vi "Create Half-H Command.vi"(8 "error in (no error)":errorcluster, 11 "Section Ptr":T8 format="%.0x") -> (0 "error out":errorcluster, 3 "Parent Ref out":T8 format="%.0x")   [LabVIEW 2015, in "DCM System Explorer.lvlib"]
uses:
  DCM System Explorer.lvlib
  <vilib>/NI Veristand/Custom Device API/Custom Device Item Ref.ctl
  <vilib>/Powertrain Controls/Device Drivers/DCM/HH/RT/Setup.ctl
  <vilib>/Powertrain Controls/Device Drivers/DCM/HH/FPGA/Mode.ctl
  <vilib>/Powertrain Controls/Device Drivers/DCM/Rev0/FPGA/Digital Channel.ctl
  <vilib>/Powertrain Controls/Device Drivers/DCM/HH/RT/Angle Control.ctl
  <vilib>/Powertrain Controls/Device Drivers/DCM/HH/RT/Config.ctl
  <vilib>/Powertrain Controls/Device Drivers/DCM/HH/RT/Mode.ctl
  <vilib>/Powertrain Controls/Device Drivers/DCM/HH/RT/ISeq.ctl
  <vilib>/NI Veristand/Custom Device API/Custom Device Channel Type.ctl
  Shared/DCM Constants and GUIDs.vi
  Shared/DCM Properties.vi
  <vilib>/NI VeriStand/Custom Device API/Custom Device API.lvlib
  DCM Shared.lvlib
  <vilib>/Powertrain Controls/Device Drivers/DCM/HH/RT/DCM - RT - HH.lvlib
  <vilib>/Powertrain Controls/Device Drivers/DCM/Rev0/FPGA/DCM - FPGA.lvlib
  <vilib>/Powertrain Controls/Device Drivers/DCM/HH/FPGA/DCM - FPGA - HH.lvlib
panel:
  in  "Config":T1[](array[typedef]) {"ISeq"."Duration [s]" min=0 max=26 format="%#_3p"; "ISeq"."Lower [A]" min=0 max=8 format="%#_3p"; "ISeq"."Upper [A]" min=0 max=8 format="%#_3p"}
  in  "Command":T4[](array[typedef])=[{"Mode"=enum."Off", "Digital Input"=enum."Unused", "Polarity"=FALSE, "Frequency [Hz]"=0.0, "Duty Cycle [%]"=0.0, "TDC Offset [CAD]"=0.0, "Window Start [DBTDC]"=0.0, "Window End [DBTDC]"=0.0, "Angles"=[{"Enable"=FALSE, "Location [DBTDC]"=0.0, "Duration [s]"=0.0}, {"Enable"=FALSE, "Location [DBTDC]"=0.0, "Duration [s]"=0.0}, {"Enable"=FALSE, "Location [DBTDC]"=0.0, "Duration [s]"=0.0}, {"Enable"=FALSE, "Location [DBTDC]"=0.0, "Duration [s]"=0.0}], "Skip Fire"=FALSE, "Skip Fire Index"=0}, {"Mode"=enum."Off", "Digital Input"=enum."Unused", "Polarity"=FALSE, "Frequency [Hz]"=0.0, "Duty Cycle [%]"=0.0, "TDC Offset [CAD]"=0.0, "Window Start [DBTDC]"=0.0, "Window End [DBTDC]"=0.0, "Angles"=[{"Enable"=FALSE, "Location [DBTDC]"=0.0, "Duration [s]"=0.0}, {"Enable"=FALSE, "Location [DBTDC]"=0.0, "Duration [s]"=0.0}, {"Enable"=FALSE, "Location [DBTDC]"=0.0, "Duration [s]"=0.0}, {"Enable"=FALSE, "Location [DBTDC]"=0.0, "Duration [s]"=0.0}], "Skip Fire"=FALSE, "Skip Fire Index"=0}, {"Mode"=enum."Off", "Digital Input"=enum."Unused", "Polarity"=FALSE, "Frequency [Hz]"=0.0, "Duty Cycle [%]"=0.0, "TDC Offset [CAD]"=0.0, "Window Start [DBTDC]"=0.0, "Window End [DBTDC]"=0.0, "Angles"=[{"Enable"=FALSE, "Location [DBTDC]"=0.0, "Duration [s]"=0.0}, {"Enable"=FALSE, "Location [DBTDC]"=0.0, "Duration [s]"=0.0}, {"Enable"=FALSE, "Location [DBTDC]"=0.0, "Duration [s]"=0.0}, {"Enable"=FALSE, "Location [DBTDC]"=0.0, "Duration [s]"=0.0}], "Skip Fire"=FALSE, "Skip Fire Index"=0}, {"Mode"=enum."Off", "Digital Input"=enum."Unused", "Polarity"=FALSE, "Frequency [Hz]"=0.0, "Duty Cycle [%]"=0.0, "TDC Offset [CAD]"=0.0, "Window Start [DBTDC]"=0.0, "Window End [DBTDC]"=0.0, "Angles"=[{"Enable"=FALSE, "Location [DBTDC]"=0.0, "Duration [s]"=0.0}, {"Enable"=FALSE, "Location [DBTDC]"=0.0, "Duration [s]"=0.0}, {"Enable"=FALSE, "Location [DBTDC]"=0.0, "Duration [s]"=0.0}, {"Enable"=FALSE, "Location [DBTDC]"=0.0, "Duration [s]"=0.0}], "Skip Fire"=FALSE, "Skip Fire Index"=0}, {"Mode"=enum."Off", "Digital Input"=enum."Unused", "Polarity"=FALSE, "Frequency [Hz]"=0.0, "Duty Cycle [%]"=0.0, "TDC Offset [CAD]"=0.0, "Window Start [DBTDC]"=0.0, "Window End [DBTDC]"=0.0, "Angles"=[{"Enable"=FALSE, "Location [DBTDC]"=0.0, "Duration [s]"=0.0}, {"Enable"=FALSE, "Location [DBTDC]"=0.0, "Duration [s]"=0.0}, {"Enable"=FALSE, "Location [DBTDC]"=0.0, "Duration [s]"=0.0}, {"Enable"=FALSE, "Location [DBTDC]"=0.0, "Duration [s]"=0.0}], "Skip Fire"=FALSE, "Skip Fire Index"=0}, {"Mode"=enum."Off", "Digital Input"=enum."Unused", "Polarity"=FALSE, "Frequency [Hz]"=0.0, "Duty Cycle [%]"=0.0, "TDC Offset [CAD]"=0.0, "Window Start [DBTDC]"=0.0, "Window End [DBTDC]"=0.0, "Angles"=[{"Enable"=FALSE, "Location [DBTDC]"=0.0, "Duration [s]"=0.0}, {"Enable"=FALSE, "Location [DBTDC]"=0.0, "Duration [s]"=0.0}, {"Enable"=FALSE, "Location [DBTDC]"=0.0, "Duration [s]"=0.0}, {"Enable"=FALSE, "Location [DBTDC]"=0.0, "Duration [s]"=0.0}], "Skip Fire"=FALSE, "Skip Fire Index"=0}, {"Mode"=enum."Off", "Digital Input"=enum."Unused", "Polarity"=FALSE, "Frequency [Hz]"=0.0, "Duty Cycle [%]"=0.0, "TDC Offset [CAD]"=0.0, "Window Start [DBTDC]"=0.0, "Window End [DBTDC]"=0.0, "Angles"=[{"Enable"=FALSE, "Location [DBTDC]"=0.0, "Duration [s]"=0.0}, {"Enable"=FALSE, "Location [DBTDC]"=0.0, "Duration [s]"=0.0}, {"Enable"=FALSE, "Location [DBTDC]"=0.0, "Duration [s]"=0.0}, {"Enable"=FALSE, "Location [DBTDC]"=0.0, "Duration [s]"=0.0}], "Skip Fire"=FALSE, "Skip Fire Index"=0}, {"Mode"=enum."Off", "Digital Input"=enum."Unused", "Polarity"=FALSE, "Frequency [Hz]"=0.0, "Duty Cycle [%]"=0.0, "TDC Offset [CAD]"=0.0, "Window Start [DBTDC]"=0.0, "Window End [DBTDC]"=0.0, "Angles"=[{"Enable"=FALSE, "Location [DBTDC]"=0.0, "Duration [s]"=0.0}, {"Enable"=FALSE, "Location [DBTDC]"=0.0, "Duration [s]"=0.0}, {"Enable"=FALSE, "Location [DBTDC]"=0.0, "Duration [s]"=0.0}, {"Enable"=FALSE, "Location [DBTDC]"=0.0, "Duration [s]"=0.0}], "Skip Fire"=FALSE, "Skip Fire Index"=0}] {"Skip Fire Index" max=7; "Angles"."Duration [s]" format="%#_3p"; "Frequency [Hz]" format="%#_3p"}
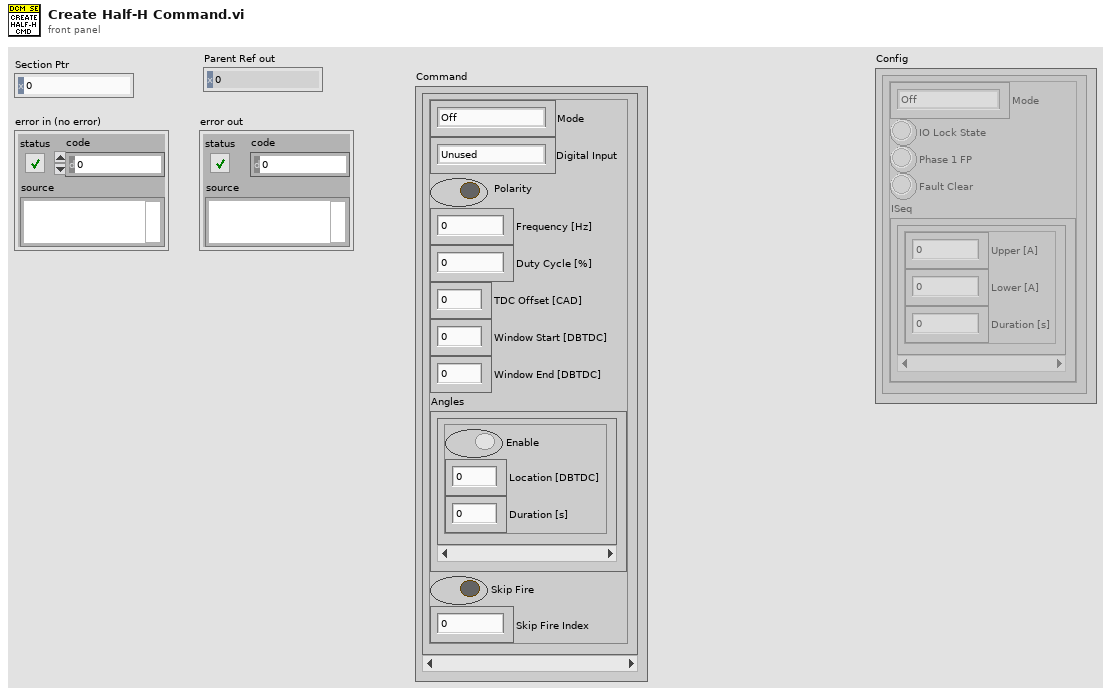
[diagram p1: front panel]
types:
  T1 = typedef "DCM - RT - HH.lvlib/Config.ctl" = cluster{"Mode":T2, "IO Lock State":bool, "Phase 1 FP":bool, "Fault Clear":bool, "ISeq":T3[]}
  T2 = typedef "DCM - RT - HH.lvlib/Mode.ctl" = enum16{"Off", "Lowside", "Highside", "PFI", "Full H", "3-Phase"}
  T3 = typedef "DCM - RT - HH.lvlib/ISeq.ctl" = cluster{"Upper [A]":sgl, "Lower [A]":sgl, "Duration [s]":sgl}
  T4 = typedef "DCM - RT - HH.lvlib/Setup.ctl" = cluster{"Mode":T5, "Digital Input":T6, "Polarity":bool, "Frequency [Hz]":sgl, "Duty Cycle [%]":sgl, "TDC Offset [CAD]":sgl, "Window Start [DBTDC]":sgl, "Window End [DBTDC]":sgl, "Angles":T7[], "Skip Fire":bool, "Skip Fire Index":u8}
  T5 = typedef "DCM - FPGA - HH.lvlib/Mode.ctl" = enum8{"Off", "Direct", "Pulse Width Modulation", "Engine Position Tracking"}
  T6 = typedef "DCM - FPGA.lvlib/Digital Channel.ctl" = enum8{"Unused", "Diff IO 1", "Diff IO 2", "Diff IO 3", "Diff IO 4", "Diff IO 5", "Diff IO 6", "Diff IO 7", "Diff IO 8", "Aux 1", "Aux 2", "Aux 3", "Aux 4", "Aux 5", "Aux 6", "Aux 7", "Aux 8", "User OS"}
  T7 = typedef "DCM - RT - HH.lvlib/Angle Control.ctl" = cluster{"Enable":bool, "Location [DBTDC]":sgl, "Duration [s]":sgl}
  T8 = typedef "Custom Device API.lvlib/Custom Device Item Ref.ctl" = u64
  T9 = typedef "Custom Device API.lvlib/Custom Device Channel Type.ctl" = enum16{"Input", "Output"}
  T10 = typedef "DCM Shared.lvlib/Channel.ctl" = cluster{"Name":string, "Units":string, "Default":dbl, "Description":string}
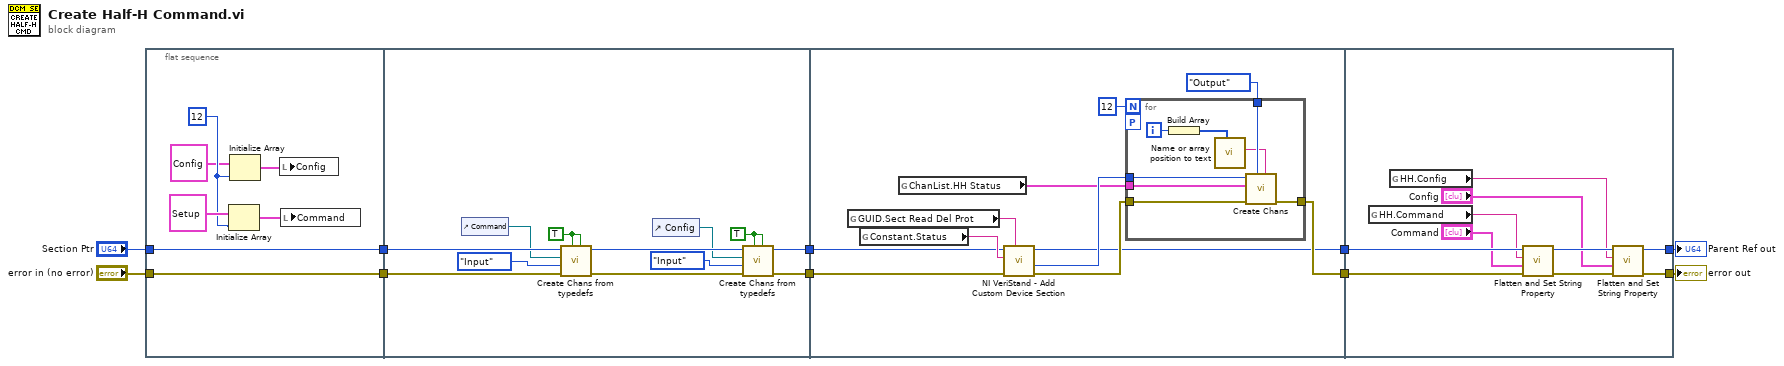
[diagram p0: block diagram]
diagram:
  n1 = flat-sequence {
    tunnel: [w16] -> w8
    tunnel: [w17] -> w9
    tunnel: "error in (no error)" -> [w17]
    tunnel: "Section Ptr" -> [w16]
    tunnel: [w23] -> w2
    tunnel: w9 -> [w20]
    tunnel: w8 -> [w21]
    tunnel: [w22] -> w4
    tunnel: w4 -> [w33]
    tunnel: [w30] -> w3
    tunnel: w2 -> [w32]
    tunnel: [w31] -> w1
    tunnel: [w49] -> w10
    tunnel: [w50] -> w5
    tunnel: w3 -> [w57]
    tunnel: w1 -> [w58]
    frame #0 {
      w13 = 12 ("dimension size")
      n2 = Initialize Array(T4 {"Mode"=enum."Off", "Digital Input"=enum."Unused", "Polarity"=FALSE, "Frequency [Hz]"=0.0, "Duty Cycle [%]"=0.0, "TDC Offset [CAD]"=0.0, "Window Start [DBTDC]"=0.0, "Window End [DBTDC]"=0.0, "Angles"=[{"Enable"=FALSE, "Location [DBTDC]"=0.0, "Duration [s]"=0.0}, {"Enable"=FALSE, "Location [DBTDC]"=0.0, "Duration [s]"=0.0}, {"Enable"=FALSE, "Location [DBTDC]"=0.0, "Duration [s]"=0.0}, {"Enable"=FALSE, "Location [DBTDC]"=0.0, "Duration [s]"=0.0}], "Skip Fire"=FALSE, "Skip Fire Index"=0}, w13) -> (w14:T4[])
      n3 = Initialize Array(T1 {"Mode"=enum."Off", "IO Lock State"=FALSE, "Phase 1 FP"=FALSE, "Fault Clear"=FALSE, "ISeq"=[{"Upper [A]"=0.0, "Lower [A]"=0.0, "Duration [s]"=0.0}, {"Upper [A]"=0.0, "Lower [A]"=0.0, "Duration [s]"=0.0}, {"Upper [A]"=0.0, "Lower [A]"=0.0, "Duration [s]"=0.0}, {"Upper [A]"=0.0, "Lower [A]"=0.0, "Duration [s]"=0.0}]} ("HH Config"), w13) -> (w11:T1[])
      n4 = local write "Config"(w11) -> ()
      n5 = local write "Command"(w14) -> ()
    }
    frame #1 {
      w27 = TRUE ("Prevent overwrite? (F)")
      w28 = TRUE ("Prevent overwrite? (F)")
      n6 = control-ref of="Command"() -> (w18:refnum<vi>)
      n7 = call "Create Chans from typedefs.vi"("Default from text? (F)"=w28, "Prevent overwrite? (F)"=w28, "error in"=w20, "Type"=Custom_Device_Channel_Type."Input", "Ctl Ref"=w18, "Section Ref in"=w21) -> ("error out"=w24:errorcluster, "Section Ref out"=w25:T8)  [unwired: 3 in, 1 out]
      n8 = control-ref of="Config"() -> (w19:refnum<vi>)
      n9 = call "Create Chans from typedefs.vi"("Default from text? (F)"=w27, "Prevent overwrite? (F)"=w27, "error in"=w24, "Type"=Custom_Device_Channel_Type."Input", "Ctl Ref"=w19, "Section Ref in"=w25) -> ("error out"=w23:errorcluster, "Section Ref out"=w22:T8)  [unwired: 3 in, 1 out]
    }
    frame #2 {
      n10 = global read "DCM Constants and GUIDs.vi" "GUID.Sect Read Del Prot"() -> (w39:string)
      n11 = global read "DCM Constants and GUIDs.vi" "Constant.Status"() -> (w38:string)
      n12 = global read "DCM Constants and GUIDs.vi" "ChanList.HH Status"() -> (w35:T10[])
      n13 = call <vilib>:"NI VeriStand - Add Custom Device Section.vi"("GUID (Default Section)"=w39, "error in (no error)"=w32, "Section Name"=w38, "Parent Ref in"=w33) -> ("error out"=w36:errorcluster, "Section Ptr"=w37:T8, "Parent Ref out"=w30:T8)  [unwired: 4 in, 1 out]
      n14 = for {
        N: 12 -> [_]
        tunnel: Custom_Device_Channel_Type."Output" ("Type") -> [w48]
        tunnel: w35 -> [w47]
        tunnel: w37 -> [w42]
        workers-P: _ -> [_]
        tunnel: w36 -> [w43]
        tunnel: [w41] -> w31
        i -> [w45]
        n15 = Build Array(w45) -> (w44:i32[])
        n16 = call "Name or array position to text.vi"("Array Positions (none)"=w44) -> ("Name out"=w46:string)  [unwired: 10 in]
        n17 = call "Create Chans.vi"("New Section Name (none)"=w46, "Type"=w48, "error in (no error)"=w43, "Channels"=w47, "Section Ptr"=w42) -> ("error out"=w41:errorcluster)  [unwired: 3 in, 3 out]
      }
    }
    frame #3 {
      n18 = global read "DCM Properties.vi" "HH.Command"() -> (w56:string)
      n19 = global read "DCM Properties.vi" "HH.Config"() -> (w52:string)
      n20 = call "Flatten and Set String Property.vi"("error in (no error)"=w58, "Value"="Command", "Property Name"=w56, "Section Ref in"=w57) -> ("error out"=w53:errorcluster, "Section Ref out"=w54:T8)  [unwired: 6 in]
      n21 = call "Flatten and Set String Property.vi"("error in (no error)"=w53, "Value"="Config", "Property Name"=w52, "Section Ref in"=w54) -> ("error out"=w49:errorcluster, "Section Ref out"=w50:T8)  [unwired: 6 in]
    }
  }
  "Parent Ref out" <- w5
  "error out" <- w10
